vi "niRFUtil MT Generate Bits.vi"(0 "total bits (128)":i32=128, 1 "mode (PN)":T4, 2 "user base bit pattern":T2 min=0, 7 "PN sequence order (9)":T3=9, 9 "seed in (0xD6BF7DF2)":T1=3602873842 format="%.0x", 11 "error in (no error)":errorcluster, 12 "base bit pattern (00001111)":T5=enum."00001111", 13 "reset? (T)":bool=TRUE) -> (4 "output bit stream":T2 min=0, 10 "seed out (PN Mode)":T1 format="%.0x", 15 "error out":errorcluster)   [LabVIEW 2015, in "niRFUtil.lvlib"]
doc: "Generates the sequence of data bits to be modulated. This VI generates bit sequences based upon a fixed pattern, a user-defined pattern, or a PN sequence. The selected pattern is repeated until the user-specified number of total bits is generated.\n\nThe VI is continuable and reentrant, meaning that after being called at least once with reset? set to TRUE, subsequent calls to the same instance of the VI generate bits that continue where the previous bit pattern left off."
uses:
  niRFUtil.lvlib
  Includes/niRFUtil INC Bit Mode.ctl
  Includes/niRFUtil INC Bit Pattern.ctl
  Includes/niRFUtil INC Bit Array.ctl
  Includes/niRFUtil INC PN Order.ctl
  Includes/niRFUtil INC PN Seed.ctl
  Utilities/niRFUtil MT UTIL GF2 Primative Poly LUT.vi
  Utilities/niRFUtil MT UTIL Calcuate PN Bits Galois.vi
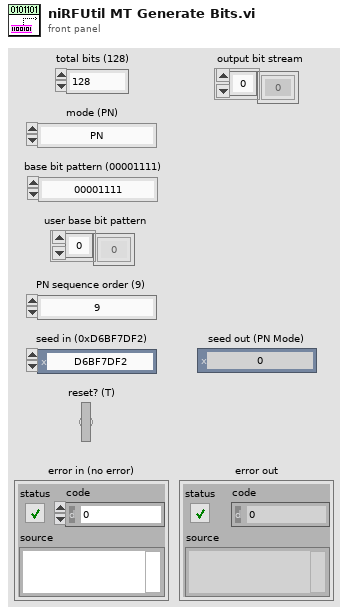
[diagram p1: front panel]
types:
  T1 = typedef "niRFUtil.lvlib/niRFUtil INC PN Seed.ctl" = u32
  T2 = typedef "niRFUtil.lvlib/niRFUtil INC Bit Array.ctl" = i8[]
  T3 = typedef "niRFUtil.lvlib/niRFUtil INC PN Order.ctl" = i32
  T4 = typedef "niRFUtil.lvlib/niRFUtil INC Bit Mode.ctl" = enum16{"PN", "pattern", "user"}
  T5 = typedef "niRFUtil.lvlib/niRFUtil INC Bit Pattern.ctl" = enum16{"0", "1", "01", "0011", "00001111"}
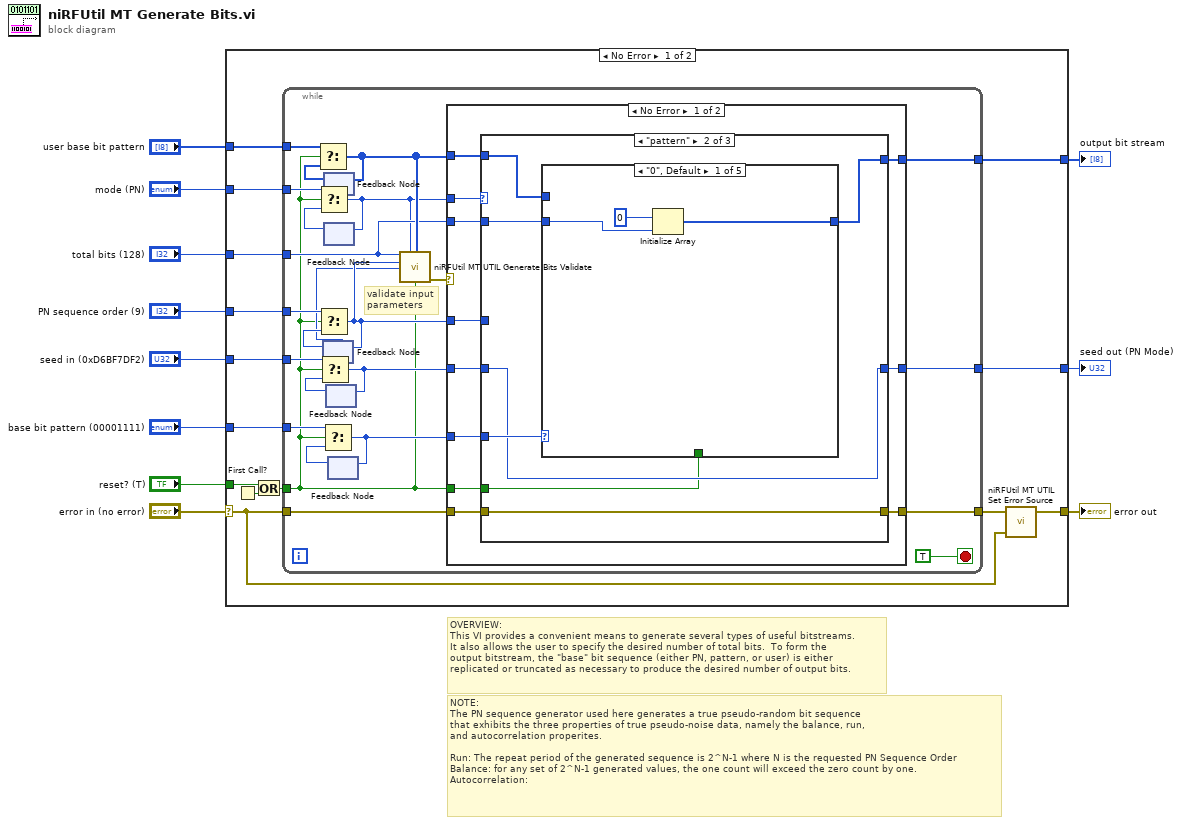
[diagram p0: block diagram]
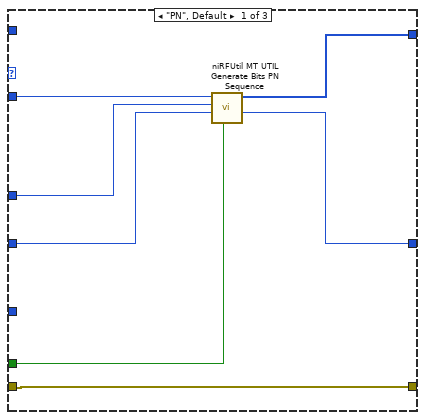
[diagram p2: hidden frame]
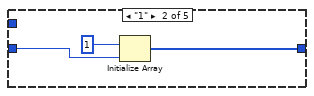
[diagram p3: hidden frame]
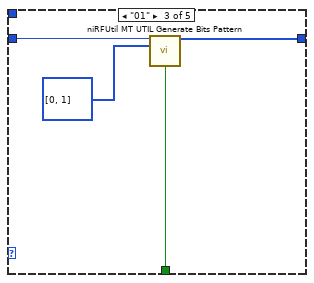
[diagram p4: hidden frame]
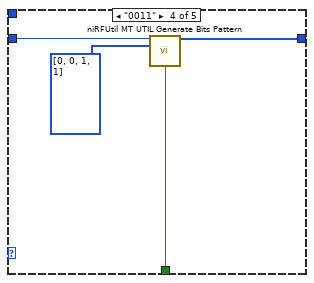
[diagram p5: hidden frame]
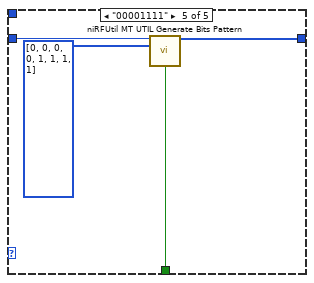
[diagram p6: hidden frame]
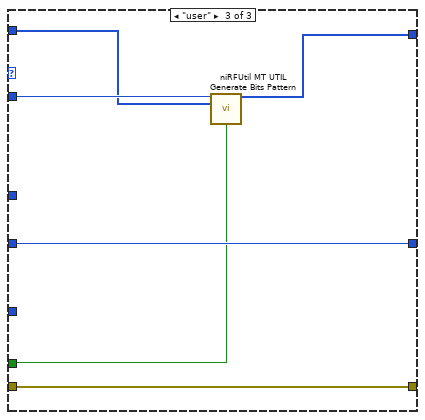
[diagram p7: hidden frame]
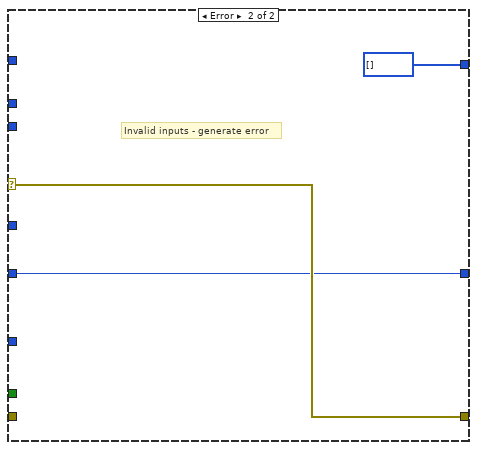
[diagram p8: hidden frame]
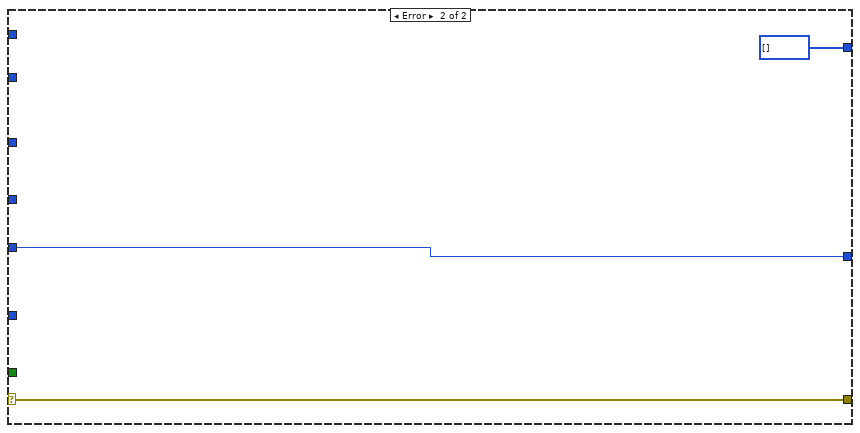
[diagram p9: hidden frame]
diagram:
  # "OVERVIEW:\nThis VI provides a convenient means to generate several types of useful bitstreams.\nIt also allows the user to specify the desired number of total bits.  To form the\noutput bitstream, the \"base\" bit sequence (either PN, pattern, or user) is either\nreplicated or truncated as necessary to produce the desired number of output bits."
  # "NOTE:\nThe PN sequence generator used here generates a true pseudo-random bit sequence\nthat exhibits the three properties of true pseudo-noise data, namely the balance, run,\nand autocorrelation properites.\n\nRun: The repeat period of the generated sequence is 2^N-1 where N is the requested PN Sequence Order\nBalance: for any set of 2^N-1 generated values, the one count will exceed the zero count by one.\nAutocorrelation:"
  n1 = case shown="No Error" "error in (no error)" {
    selector: "error in (no error)" -> [w12 w103]
    tunnel: [w18 w103] -> w10
    tunnel: "total bits (128)" -> [w23 _]
    tunnel: "mode (PN)" -> [w21 _]
    tunnel: "reset? (T)" -> [w15 _]
    tunnel: "base bit pattern (00001111)" -> [w24 _]
    tunnel: "seed in (0xD6BF7DF2)" -> [w14 w102]
    tunnel: "PN sequence order (9)" -> [w22 _]
    tunnel: [w25 i8[] []] -> w2
    tunnel: "user base bit pattern" -> [w20 _]
    tunnel: [w17 w102] -> w1
    frame No Error {
      n2 = First Call?() -> (First Call?: T/F=w16:bool)
      n3 = Or(x=w15, y=w16) -> (x .or. y?=w13:bool)
      n4 = while {
        tunnel: [w48] -> w25
        tunnel: w24 -> [w32]
        tunnel: w23 -> [w36]
        tunnel: w22 -> [w38]
        tunnel: w21 -> [w29]
        tunnel: w20 -> [w42]
        tunnel: [w46] -> w19
        tunnel: w12 -> [w45]
        tunnel: [w44] -> w17
        tunnel: w14 -> [w35]
        tunnel: w13 -> [w28]
        stop <- TRUE stop-if-true
        # "validate input parameters"
        n5 = feedback #1() -> (w39:T3)  [unwired: 1 out]
        n6 = Select(t=w38, s=w28, f=w39) -> (s? t:f=w37:T3)
        n7 = feedback-in #1(w37) -> ()
        n8 = feedback #2() -> (w43:T2)  [unwired: 1 out]
        n9 = Select(t=w42, s=w28, f=w43) -> (s? t:f=w40:T2)
        n10 = feedback-in #2(w40) -> ()
        n11 = feedback #3() -> (w27:T4)  [unwired: 1 out]
        n12 = Select(t=w29, s=w28, f=w27) -> (s? t:f=w26:T4)
        n13 = feedback-in #3(w26) -> ()
        n14 = feedback #4() -> (w34:T1)  [unwired: 1 out]
        n15 = Select(t=w35, s=w28, f=w34) -> (s? t:f=w33:T1)
        n16 = feedback-in #4(w33) -> ()
        n17 = feedback #5() -> (w31:T5)  [unwired: 1 out]
        n18 = Select(t=w32, s=w28, f=w31) -> (s? t:f=w30:T5)
        n19 = feedback-in #5(w30) -> ()
        n20 = call "niRFUtil MT UTIL Generate Bits Validate.vi"("Total Bits"=w36, "Mode (PN)"=w26, "User Base Bit Pattern"=w40, "PN Sequence Order"=w37, "seed in"=w33, "reset?"=w28) -> ("error out"=w47:errorcluster)  [unwired: 9 out]
        n21 = case shown="No Error" w47 {
          selector: w47 -> [_ w100]
          tunnel: w45 -> [w59 _]
          tunnel: [w58 w100] -> w46
          tunnel: w26 -> [w57 _]
          tunnel: [w56 i8[] [] ("Output Data Bit Sequence")] -> w48
          tunnel: w36 -> [w55 _]
          tunnel: w37 -> [w54 _]
          tunnel: w33 -> [w53 w99]
          tunnel: w30 -> [w52 _]
          tunnel: w28 -> [w51 _]
          tunnel: w40 -> [w50 _]
          tunnel: [w49 w99] -> w44
          frame No Error {
            n22 = case shown="\"pattern\"" w57 {
              tunnel: w59 -> [w61 w73 w97]
              tunnel: [w61 w73 w97] -> w58
              tunnel: w50 -> [_ w71 w95]
              tunnel: [w66 w69 w94] -> w56
              tunnel: w55 -> [w65 w70 w96]
              tunnel: w54 -> [w64 _ _]
              tunnel: w53 -> [w63 w68 w93]
              tunnel: w52 -> [_ w72 _]
              tunnel: w51 -> [w62 w67 w92]
              tunnel: [w60 w68 w93] -> w49
              frame "PN", Default {
                n23 = call "niRFUtil MT UTIL Generate Bits PN Sequence.vi"("Reset? (T)"=w62, "seed in (0xD6BF7DF2)"=w63, "PN Sequence Order (9)"=w64, "Total Bits"=w65) -> ("seed out"=w60:T1, "Output Bit Stream"=w66:T2)  [unwired: 6 out]
              }
              frame "pattern" {
                n24 = case shown="\"0\", Default" w72 {
                  tunnel: w71 -> [_ _ _ _ _]
                  tunnel: w70 -> [w75 w78 w82 w86 w90]
                  tunnel: [w74 w77 w83 w87 w91] -> w69
                  tunnel: w67 -> [_ _ w80 w84 w88]
                  frame "0", Default {
                    n25 = Initialize Array(i8 0, w75) -> (w74:i8[])
                  }
                  frame "1" {
                    n26 = Initialize Array(i8 1, w78) -> (w77:i8[])
                  }
                  frame "01" {
                    n27 = call "niRFUtil MT UTIL Generate Bits Pattern.vi"("Total Bits"=w82, "Reset? (T)"=w80, "User Base Bit Pattern"=T2 [0, 1] ("Base Bit Pattern")) -> ("Output Bit Stream"=w83:T2)  [unwired: 12 out]
                  }
                  frame "0011" {
                    n28 = call "niRFUtil MT UTIL Generate Bits Pattern.vi"("Total Bits"=w86, "Reset? (T)"=w84, "User Base Bit Pattern"=T2 [0, 0, 1, 1] ("Base Bit Pattern")) -> ("Output Bit Stream"=w87:T2)  [unwired: 12 out]
                  }
                  frame "00001111" {
                    n29 = call "niRFUtil MT UTIL Generate Bits Pattern.vi"("Total Bits"=w90, "Reset? (T)"=w88, "User Base Bit Pattern"=T2 [0, 0, 0, 0, 1, 1, 1, 1] ("Base Bit Pattern")) -> ("Output Bit Stream"=w91:T2)  [unwired: 12 out]
                  }
                }
              }
              frame "user" {
                n30 = call "niRFUtil MT UTIL Generate Bits Pattern.vi"("Total Bits"=w96, "Reset? (T)"=w92, "User Base Bit Pattern"=w95) -> ("Output Bit Stream"=w94:T2)  [unwired: 12 out]
              }
            }
          }
          frame Error {
            # "Invalid inputs - generate error"
          }
        }
      }
      n31 = call "niRFUtil MT UTIL Set Error Source.vi"("initial error in (no error)"=w12, "final error in (no error)"=w19) -> ("error out"=w18:errorcluster)  [unwired: 3 in]
    }
    frame Error {
    }
  }
  "error out" <- w10
  "output bit stream" <- w2
  "seed out (PN Mode)" <- w1
